vi "GripSensorConversion.vi"(1 "Grip Sensor Output (g)":dbl) -> (0 "Grip Force (N)":dbl)   [LabVIEW 2019]
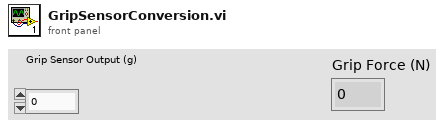
[diagram p1: front panel]
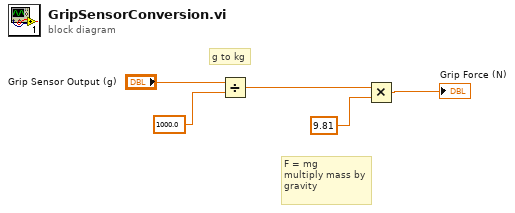
[diagram p0: block diagram]
diagram:
  # "g to kg"
  # "F = mg\nmultiply mass by gravity"
  n1 = Divide(x="Grip Sensor Output (g)", y=1000.0) -> (x/y=w3:dbl)
  n2 = Multiply(x=w3, y=9.81) -> (x*y=→"Grip Force (N)":dbl)
